vi "Find Object Item Locations by Names.vi"(5 "Insertion point if not found":bool, 6 "Only return first found":bool, 7 "Item Names <JSON>":string[](array[string]), 8 "error in (no error)":errorcluster, 10 "Object Offset":i32, 11 "JSON":string) -> (0 "error out":errorcluster, 1 "Items":T1[](array[typedef]))   [LabVIEW 2017, in "JSONtext.lvlib"]
uses:
  JSONtext.lvlib
  Parsing/Found Items.ctl
  Parsing/Parsing State.ctl
  Parsing/Advance past String.vi
  Parsing/Advance past Number.vi
  Parsing/Advance past Array.vi
  Parsing/Advance past Object.vi
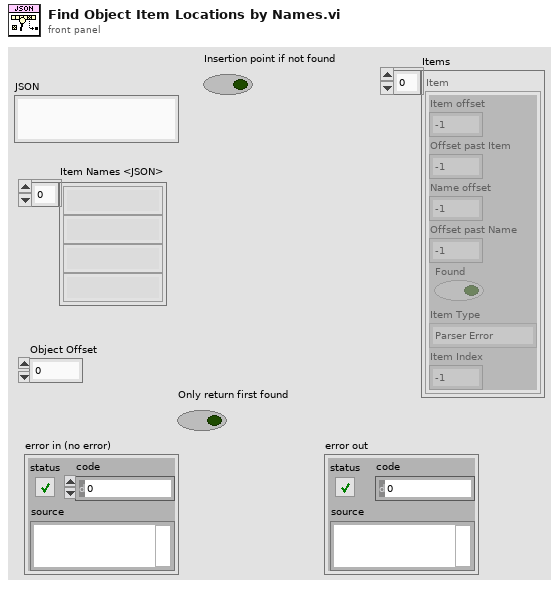
[diagram p1: front panel]
types:
  T1 = typedef "JSONtext.lvlib/Found Items.ctl" = cluster{"Item offset":i32, "Offset past Item":i32, "Name offset":i32, "Offset past Name":i32, "Found":bool, "Item Type":T2, "Item Index":i32}
  T2 = typedef "JSONtext.lvlib/Parsing State.ctl" = enum16{"Parser Error", "Object", "Array", "String", "Number/Other", "Leading Whitespace", "Object end", "Array end", "Value end"}
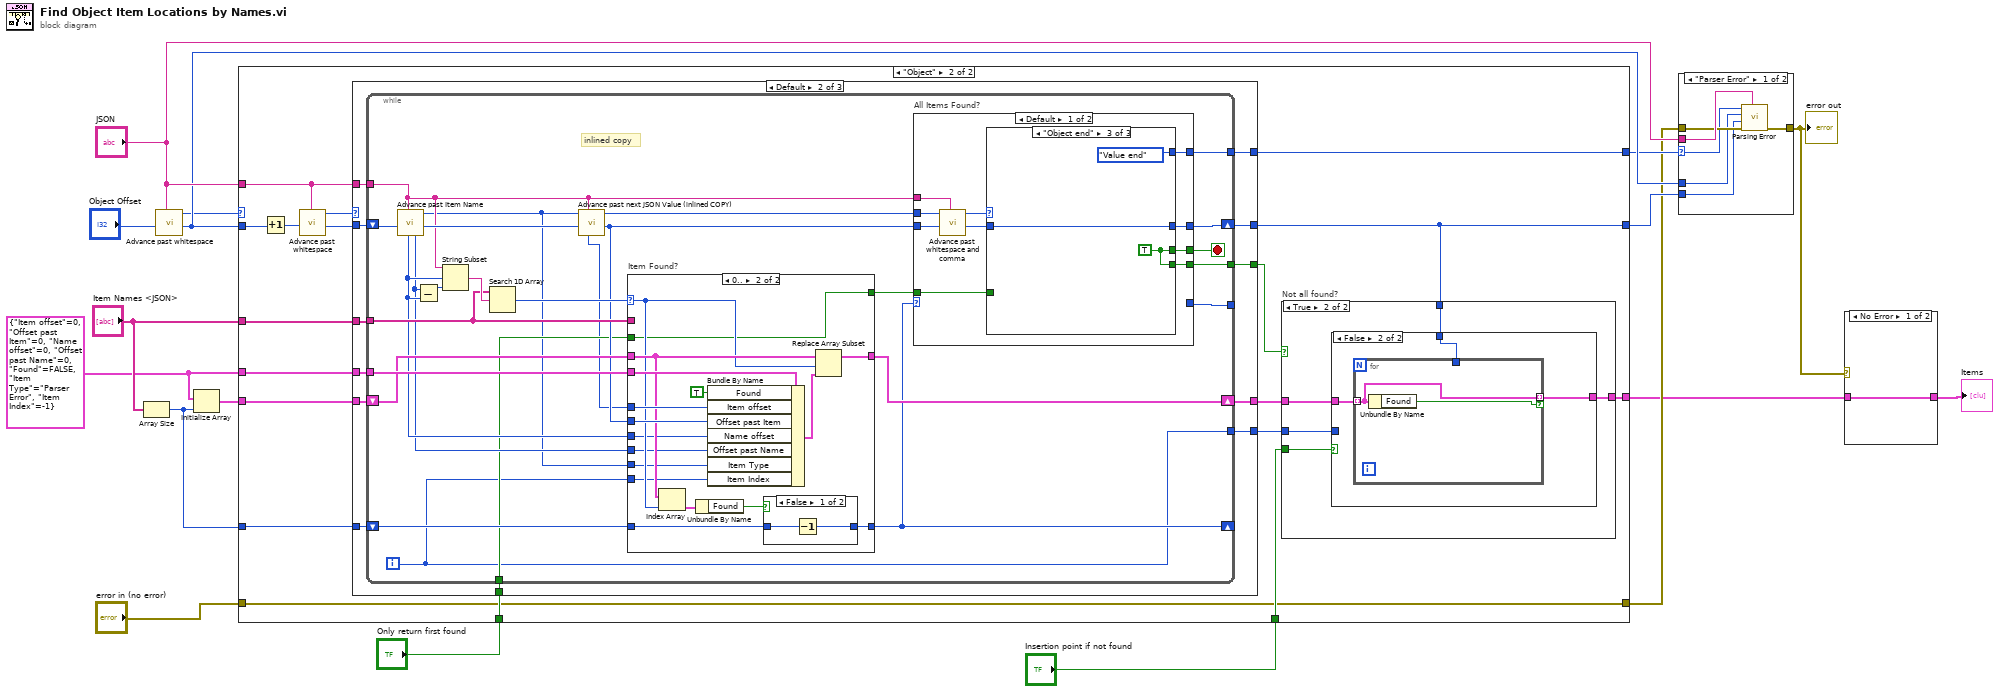
[diagram p0: block diagram]
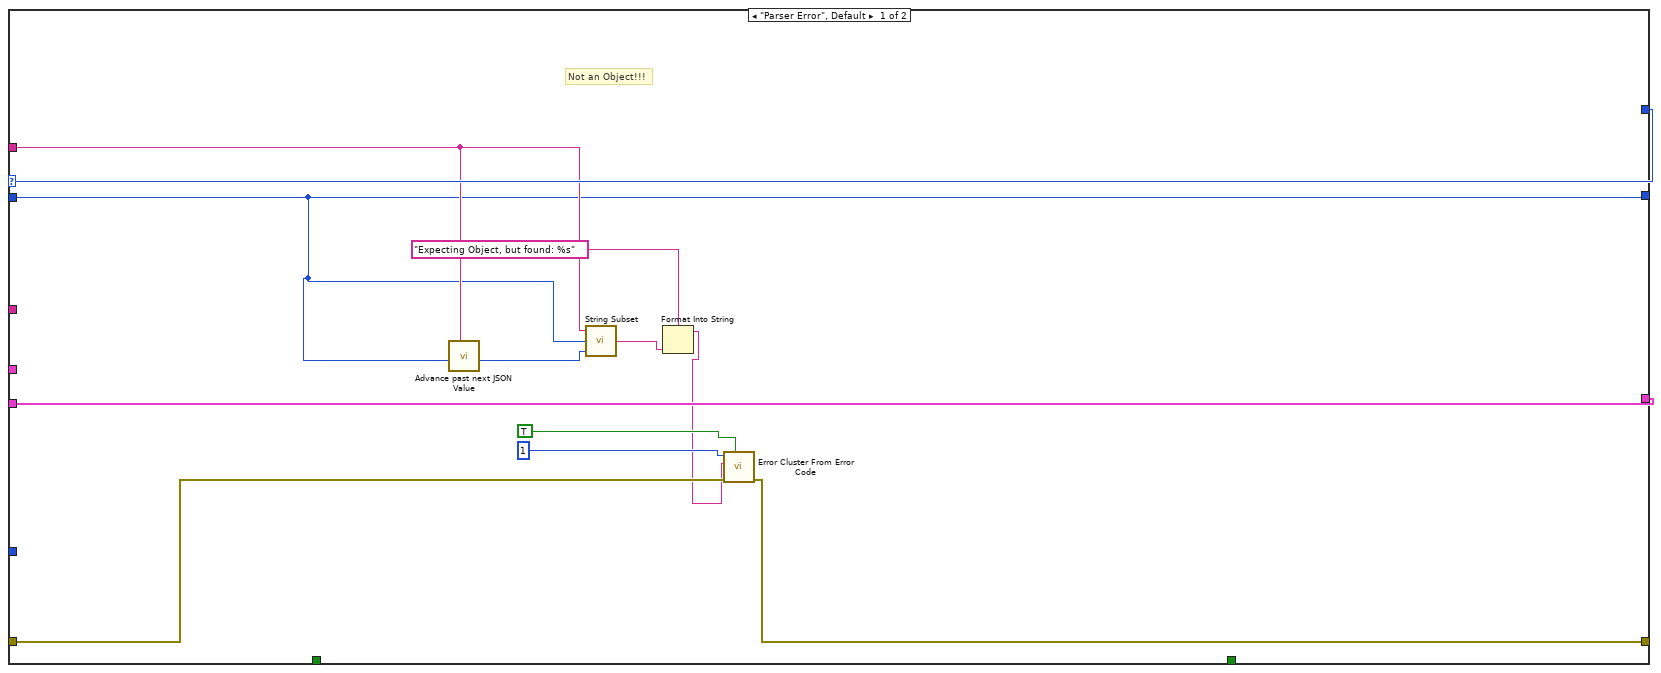
[diagram p3: hidden frame]
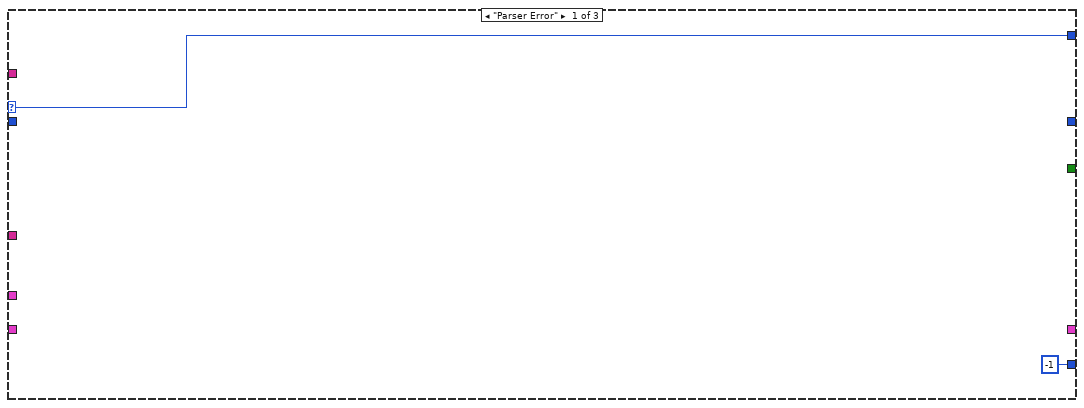
[diagram p4: hidden frame]
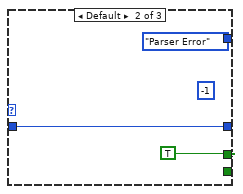
[diagram p8: hidden frame]
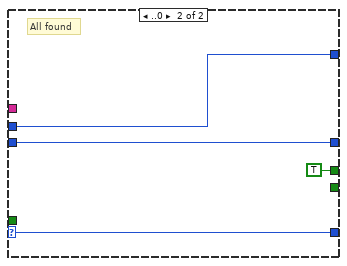
[diagram p9: hidden frame]
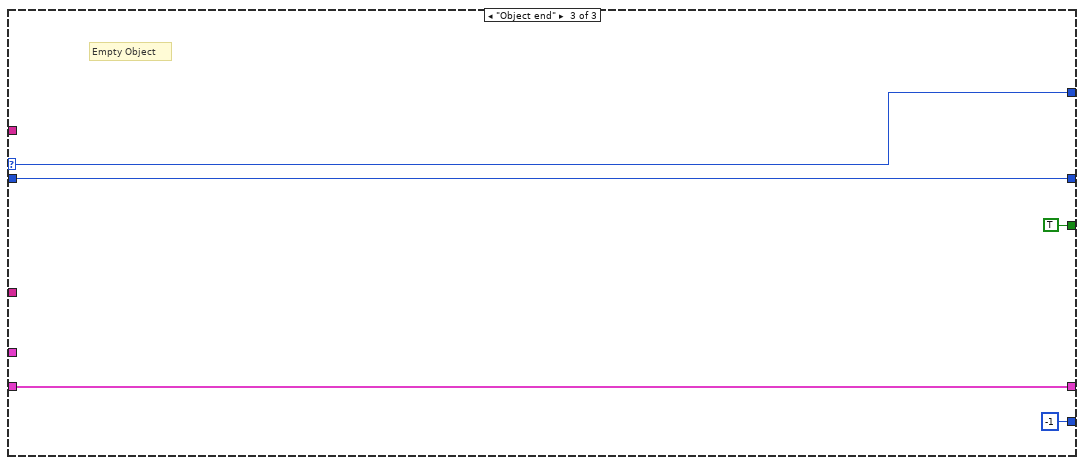
[diagram p10: hidden frame]
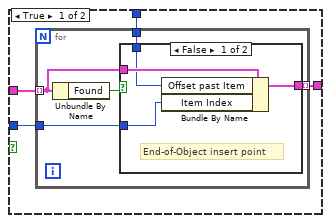
[diagram p12: hidden frame]
diagram:
  w14 = T1 {"Item offset"=0, "Offset past Item"=0, "Name offset"=0, "Offset past Name"=0, "Found"=FALSE, "Item Type"=enum."Parser Error", "Item Index"=-1}
  n1 = Array Size(array="Item Names <JSON>") -> (size(s)=w13:i32)
  n2 = call "Advance past whitespace.vi"("JSON"="JSON", "Offset"="Object Offset") -> ("Offset of first non-whitespace"=w10:i32, "Parser State"=w9:T2)  [unwired: 8 in]
  n3 = Initialize Array(w14, w13) -> (w15:T1[])
  n4 = case shown="\"Object\"" w9 {
    selector: w9 -> [w25 _]
    tunnel: "Item Names <JSON>" -> [_ w47]
    tunnel: w15 -> [w29 w46]
    tunnel: w14 -> [_ w45]
    tunnel: w13 -> [_ w44]
    tunnel: [w29 w41] -> w1
    tunnel: "JSON" -> [w20 w33]
    tunnel: [w19 w40] -> w11
    tunnel: w10 -> [w19 w39]
    tunnel: [w25 w38] -> w8
    tunnel: "Only return first found" -> [_ w37]
    tunnel: "Insertion point if not found" -> [_ w36]
    tunnel: "error in (no error)" -> [w26 w35]
    tunnel: [w23 w35] -> w4
    frame "Parser Error", Default {
      # "Not an Object!!!"
      n5 = call "Advance past next JSON Value.vi"("JSON"=w20, "Offset"=w19) -> ("Offset out"=w18:i32)  [unwired: 7 in, 2 out]
      n6 = call "String Subset.vi"("Offset past End"=w18, "Start offset"=w19, "JSON"=w20) -> ("substring"=w24:string)  [unwired: 2 in]
      n7 = Format Into String(format string="Expecting Object, but found: %s", w24) -> (resulting string=w21:string)  [unwired: 2 in, 1 out]
      n8 = call <vilib>:"Error Cluster From Error Code.vi"("show call chain? (False)"=TRUE, "error in (no error)"=w26, "error message (\"\")"=w21, "error code (0)"=1) -> ("error out"=w23:errorcluster)  [unwired: 5 in]
    }
    frame "Object" {
      n9 = Increment(x=w39) -> (x+1=w34:i32)
      n10 = call "Advance past whitespace.vi"("JSON"=w33, "Offset"=w34) -> ("Offset of first non-whitespace"=w32:i32, "Parser State"=w31:T2)  [unwired: 8 in]
      n11 = case shown="Default" w31 {
        selector: w31 -> [w49 _ w136]
        tunnel: w32 -> [_ w61 w135]
        tunnel: w47 -> [_ w60 _]
        tunnel: w46 -> [_ w59 w134]
        tunnel: w45 -> [_ w58 _]
        tunnel: w44 -> [_ w57 _]
        tunnel: [_ w56 w134] -> w43
        tunnel: [_ w55 TRUE] -> w42
        tunnel: w33 -> [_ w54 _]
        tunnel: [_ w53 w135] -> w40
        tunnel: [w49 w52 w136] -> w38
        tunnel: w37 -> [_ w51 _]
        tunnel: [-1 w50 -1] -> w30
        frame "Parser Error" {
        }
        frame Default {
          n12 = while {
            shift-right: [w87] -> w53
            shift-left: w61 -> [w84]
            tunnel: w54 -> [w81]
            tunnel: [w85] -> w52
            tunnel: w60 -> [w75]
            tunnel: [w79] -> _
            tunnel: w58 -> [w77]
            shift-right: [w73] -> w56
            shift-left: w59 -> [w74]
            shift-right: [w71] -> _
            shift-left: w57 -> [w72]
            tunnel: [w69] -> w55
            tunnel: w51 -> [w66]
            tunnel: [w62] -> w50
            i -> [w62]
            stop <- w86 stop-if-true
            # "inlined copy"
            n13 = call "Advance past Item Name.vi"("JSON"=w81, "Offset"=w84) -> ("Offset past colon"=w82:i32, "State"=w63:T2, "Offset past Name"=w67:i32, "Name start out"=w68:i32)  [unwired: 6 in]
            n14 = Subtract(x=w67, y=w68) -> (x-y=w80:i32)
            n15 = String Subset(string=w81, offset (0)=w68, length (rest)=w80) -> (substring=w78:string)
            n16 = Search 1D Array(1D array=w75, element=w78) -> (index of element=w76:i32)  [unwired: 1 in]
            n17 = call "Advance past next JSON Value (inlined COPY).vi"("JSON"=w81, "Offset"=w82, "State"=w63) -> ("Offset"=w70:i32, "State"=w83:T2, "Value start"=w64:i32)  [unwired: 4 in, 2 out]
            n18 = case "Item Found?" shown="0.." w76 {
              selector: w76 -> [_ w100]
              tunnel: w77 -> [_ w106]
              tunnel: w64 -> [_ w104]
              tunnel: w70 -> [_ w103]
              tunnel: w75 -> [_ _]
              tunnel: w74 -> [w89 w101]
              tunnel: [w89 w99] -> w73
              tunnel: w72 -> [w88 w96]
              tunnel: [w88 w95] -> w71
              tunnel: w68 -> [_ w94]
              tunnel: w67 -> [_ w93]
              tunnel: w66 -> [_ w92]
              tunnel: [_ w92] -> w65
              tunnel: w63 -> [_ w91]
              tunnel: w62 -> [_ w90]
              frame Default {
              }
              frame 0.. {
                n19 = Index Array(array=w101, index=w100) -> (element=w98:T1)
                n20 = Unbundle By Name(w98) -> ("Found"=w97:bool)
                n21 = Bundle By Name(cluster=w106, "Found"=TRUE, "Item offset"=w104, "Offset past Item"=w103, "Name offset"=w94, "Offset past Name"=w93, "Item Type"=w91, "Item Index"=w90) -> (w102:T1)
                n22 = case shown="False" w97 {
                  tunnel: w96 -> [w108 w109]
                  tunnel: [w107 w109] -> w95
                  frame False {
                    n23 = Decrement(x=w108) -> (x-1=w107:i32)
                  }
                  frame True {
                  }
                }
                n24 = Replace Array Subset(array=w101, new element=w102, index=w100) -> (w99:T1[])
              }
            }
            n25 = case "All Items Found?" shown="Default" w71 {
              selector: w71 -> [_ w129]
              tunnel: [w118 w131] -> w87
              tunnel: [w117 TRUE] -> w86
              tunnel: [w116 w132] -> w85
              tunnel: w83 -> [w111 w132]
              tunnel: w70 -> [w114 w131]
              tunnel: w81 -> [w115 _]
              tunnel: [_ w129] -> w79
              tunnel: [w112 _] -> w69
              tunnel: w65 -> [w110 _]
              frame Default {
                n26 = call "Advance past whitespace and comma.vi"("JSON"=w115, "Offset"=w114, "State in"=w111) -> ("Offset past match"=w113:i32, "State"=w119:T2)  [unwired: 7 in]
                n27 = case shown="\"Object end\"" w119 {
                  selector: w119 -> [w120 _ _]
                  tunnel: [w121 TRUE w127] -> w117
                  tunnel: [w120 Parsing_State."Parser Error" Parsing_State."Value end"] -> w116
                  tunnel: w113 -> [w122 w123 w126]
                  tunnel: [w122 w123 w126] -> w118
                  tunnel: [_ _ w127] -> w112
                  tunnel: w110 -> [w121 _ _]
                  frame "Object".."Number/Other" {
                  }
                  frame Default {
                    (unwired) -1 ("Item start")
                  }
                  frame "Object end" {
                    w127 = TRUE
                  }
                }
              }
              frame ..0 {
                # "All found"
              }
            }
          }
        }
        frame "Object end" {
          # "Empty Object"
        }
      }
      n28 = case "Not all found?" shown="True" w42 {
        tunnel: w43 -> [w138 w143]
        tunnel: [w138 w142] -> w41
        tunnel: w40 -> [_ w141]
        tunnel: w36 -> [_ w140]
        tunnel: w30 -> [_ w139]
        frame False {
        }
        frame True {
          n29 = case shown="False" w140 {
            tunnel: w143 -> [w148 w161]
            tunnel: [w147 w160] -> w142
            tunnel: w141 -> [w146 w159]
            tunnel: w139 -> [w145 _]
            frame True {
              n30 = Increment(x=w145) -> (x+1=w144:i32)
              n31 = for {
                tunnel: w148 -> [w151] mode=indexing
                tunnel: [w152] -> w147 mode=indexing
                tunnel: w146 -> [w150]
                tunnel: w144 -> [w149]
                n32 = Unbundle By Name(w151) -> ("Found"=w153:bool)
                n33 = case shown="False" w153 {
                  tunnel: [w156 w158] -> w152
                  tunnel: w151 -> [w157 w158]
                  tunnel: w150 -> [w155 _]
                  tunnel: w149 -> [w154 _]
                  frame False {
                    # "End-of-Object insert point"
                    n34 = Bundle By Name(cluster=w157, "Offset past Item"=w155, "Item Index"=w154) -> (w156:T1)
                  }
                  frame True {
                  }
                }
              }
            }
            frame False {
              n35 = for {
                tunnel: w161 -> [w163] mode=indexing
                tunnel: [w163] -> w160 mode=indexing if=w162
                tunnel: w159 -> [_]
                n36 = Unbundle By Name(w163) -> ("Found"=w162:bool)
              }
            }
          }
        }
      }
    }
  }
  n37 = case shown="\"Parser Error\"" w8 {
    selector: w8 -> [w164 _]
    tunnel: "JSON" -> [w169 _]
    tunnel: w4 -> [w168 w170]
    tunnel: [w167 w170] -> w3
    tunnel: w10 -> [w166 _]
    tunnel: w11 -> [w165 _]
    frame "Parser Error" {
      n38 = call "Parsing Error.vi"("JSON"=w169, "error in (no error)"=w168, "Offset past match"=w165, "Value start"=w166, "State"=w164) -> ("error out"=w167:errorcluster)  [unwired: 6 in]
    }
    frame Default {
    }
  }
  "error out" <- w3
  n39 = case shown="No Error" w3 {
    tunnel: [w171 _] -> w2
    tunnel: w1 -> [w171 _]
    frame No Error {
    }
    frame Error {
    }
  }
  "Items" <- w2
